vi "Touch.vi"   [LabVIEW 2016, in "EV3Group10.lvrbt"]
uses:
  EV3Group10.lvrbt
  <vilib>/NXT/Block Support/NXT_InputPort.ctl
  <vilib>/NXT/Block Support/NXT_OutputPort.ctl
  <vilib>/NXT/NXTIO Xnodes/NXTIONodeSubVIs/NXTMoveMotors.vi
  <vilib>/NXT/NXTIO Xnodes/NXTIONodeSubVIs/NXTStopMotors.vi
  <vilib>/NXT/Subs/LVHSConnector.ctl
  <vilib>/NXT/NXTIO Xnodes/AddressXNode/NXTIOAddress.xnode
  <vilib>/NXT/NXTIO Xnodes/NXTIOXNode/NXTIO.xnode
  <vilib>/NXT/LegoClasses/BrickReference/BrickReference.lvclass
types:
  T1 = typedef "NXT_InputPort.ctl" = u32
  T2 = typedef "NXT_OutputPort.ctl" = u8
  T3 = typedef "LVHSConnector.ctl" = refnum<class "BrickReference.lvclass">
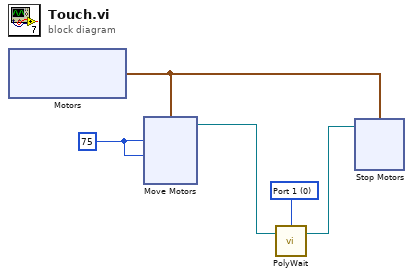
[diagram p0: block diagram]
diagram:
  w1 = i8 75 ("Power/Speed 1")
  w4 = T1 0 items=["Port 1", "Port 2", "Port 3", "Port 4"] ("Port (Port 1)")
  n1 = xnode "Motors"() -> ("Motor"=w5:cluster{"Port":T2, "Port":T2})
  n2 = xnode "Move Motors"("Power/Speed 2"=w1, "Power/Speed 1"=w1, "Motors"=w5) -> ("NXT/EV3"=w3:T3)  [unwired: 1 in]
  n3 = call-poly <vilib>:"PolyWait.vi"("NXT/EV3"=w3, "Port (Port 1)"=w4) -> ("NXT/EV3"=w2:T3)  [unwired: 2 in]
  n4 = xnode "Stop Motors"("Motors"=w5, "NXT/EV3"=w2) -> ()  [unwired: 1 out]
